vi "picoquant_close_device_handle.vi"(8 "error in (no error)":errorcluster, 11 "picoharp in":refnum<class "picoharp.lvclass">) -> (0 "error out":errorcluster, 3 "picoharp out":refnum<class "picoharp.lvclass">)   [LabVIEW 2015, in "picoharp.lvclass"]
uses:
  picoharp.lvclass
  picoharp.lvclass/picoharp.ctl
  phlib.dll
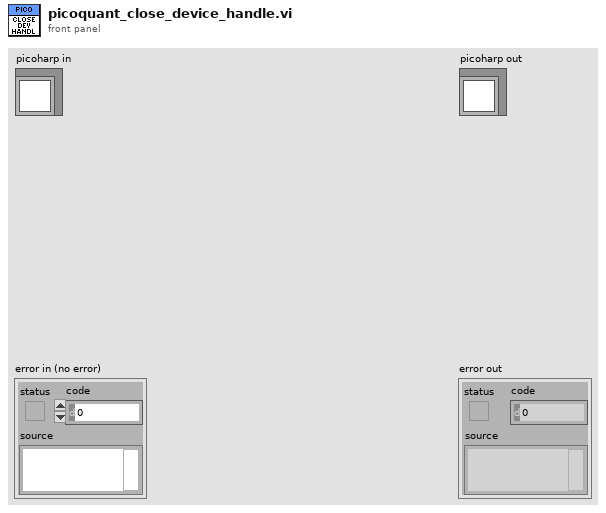
[diagram p1: front panel]
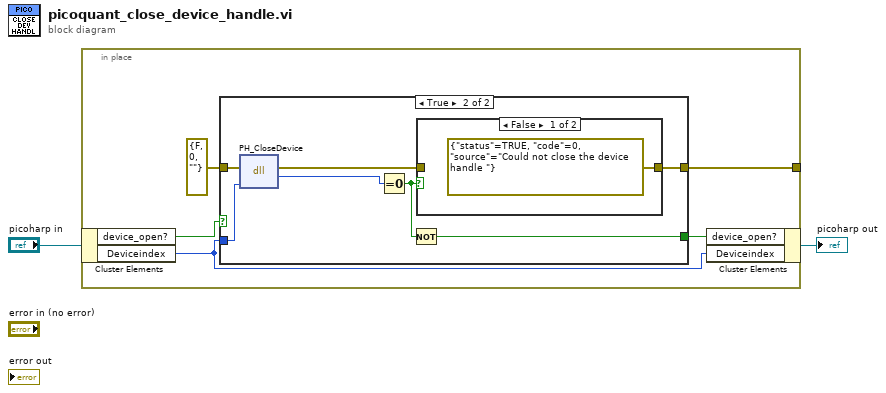
[diagram p0: block diagram]
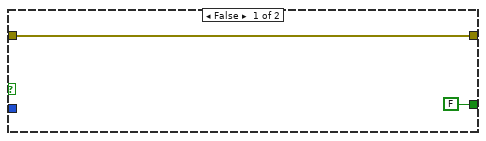
[diagram p2: hidden frame]
diagram:
  n1 = in-place {
    in-place-border: [w5] -> _
    n2 = in-place-cluster #1("picoharp in") -> ("device_open?"=w7:bool, "Deviceindex"=w6:i32)
    n3 = case shown="True" w7 {
      tunnel: w6 -> [_ w16]
      tunnel: errorcluster {"status"=FALSE, "code"=0, "source"=""} ("error in (no error)") -> [w9 w15]
      tunnel: [w9 w11] -> w5
      tunnel: [FALSE w14] -> w4
      frame False {
      }
      frame True {
        n4 = dll-call lib="phlib.dll" fn="PH_CloseDevice"(error in=w15, "devidx"=w16) -> (error out=w12:errorcluster, "return type"=w10:i32)  [unwired: 3 in, 1 out]
        n5 = Equal To 0?(x=w10) -> (x = 0?=w13:bool)
        n6 = Not(x=w13) -> (.not. x?=w14:bool)
        n7 = case shown="False" w13 {
          tunnel: w12 -> [_ w18]
          tunnel: [errorcluster {"status"=TRUE, "code"=0, "source"="Could not close the device handle "} ("error out") w18] -> w11
          frame False {
          }
          frame True {
          }
        }
      }
    }
    n8 = in-place-cluster #1("device_open?"=w4, "Deviceindex"=w6) -> (→"picoharp out":refnum<class "picoharp.lvclass">)
  }
